vi "kalman transmit and receive state updates.vi"(7 "min photons to update":u32, 8 "update z":bool, 9 "update y":bool, 10 "update x":bool, 11 "3-axis PV tracking state":T2) -> (0 "Timed Out?":bool, 2 "num kalmans queued":u16, 3 "3-axis PV tracking state out":T2, 4 "kalman to host":cluster{"Kalman State":T1, "Kalman Update":bool})   [LabVIEW 2010]
uses:
  kalman 3-axis state.ctl
  integrating single axis kalman state.ctl
  <vilib>/rvi/DataTransferAndStorage/Container/XNode/niFpgaContainer.xnode
  <vilib>/rvi/FIFO/Fifo_Resource/nirvififoEmulationSetSize.vi
  <vilib>/rvi/DataTransferAndStorage/Container/Common/niFpgaContainerGetUniqueNameForEmu.vi
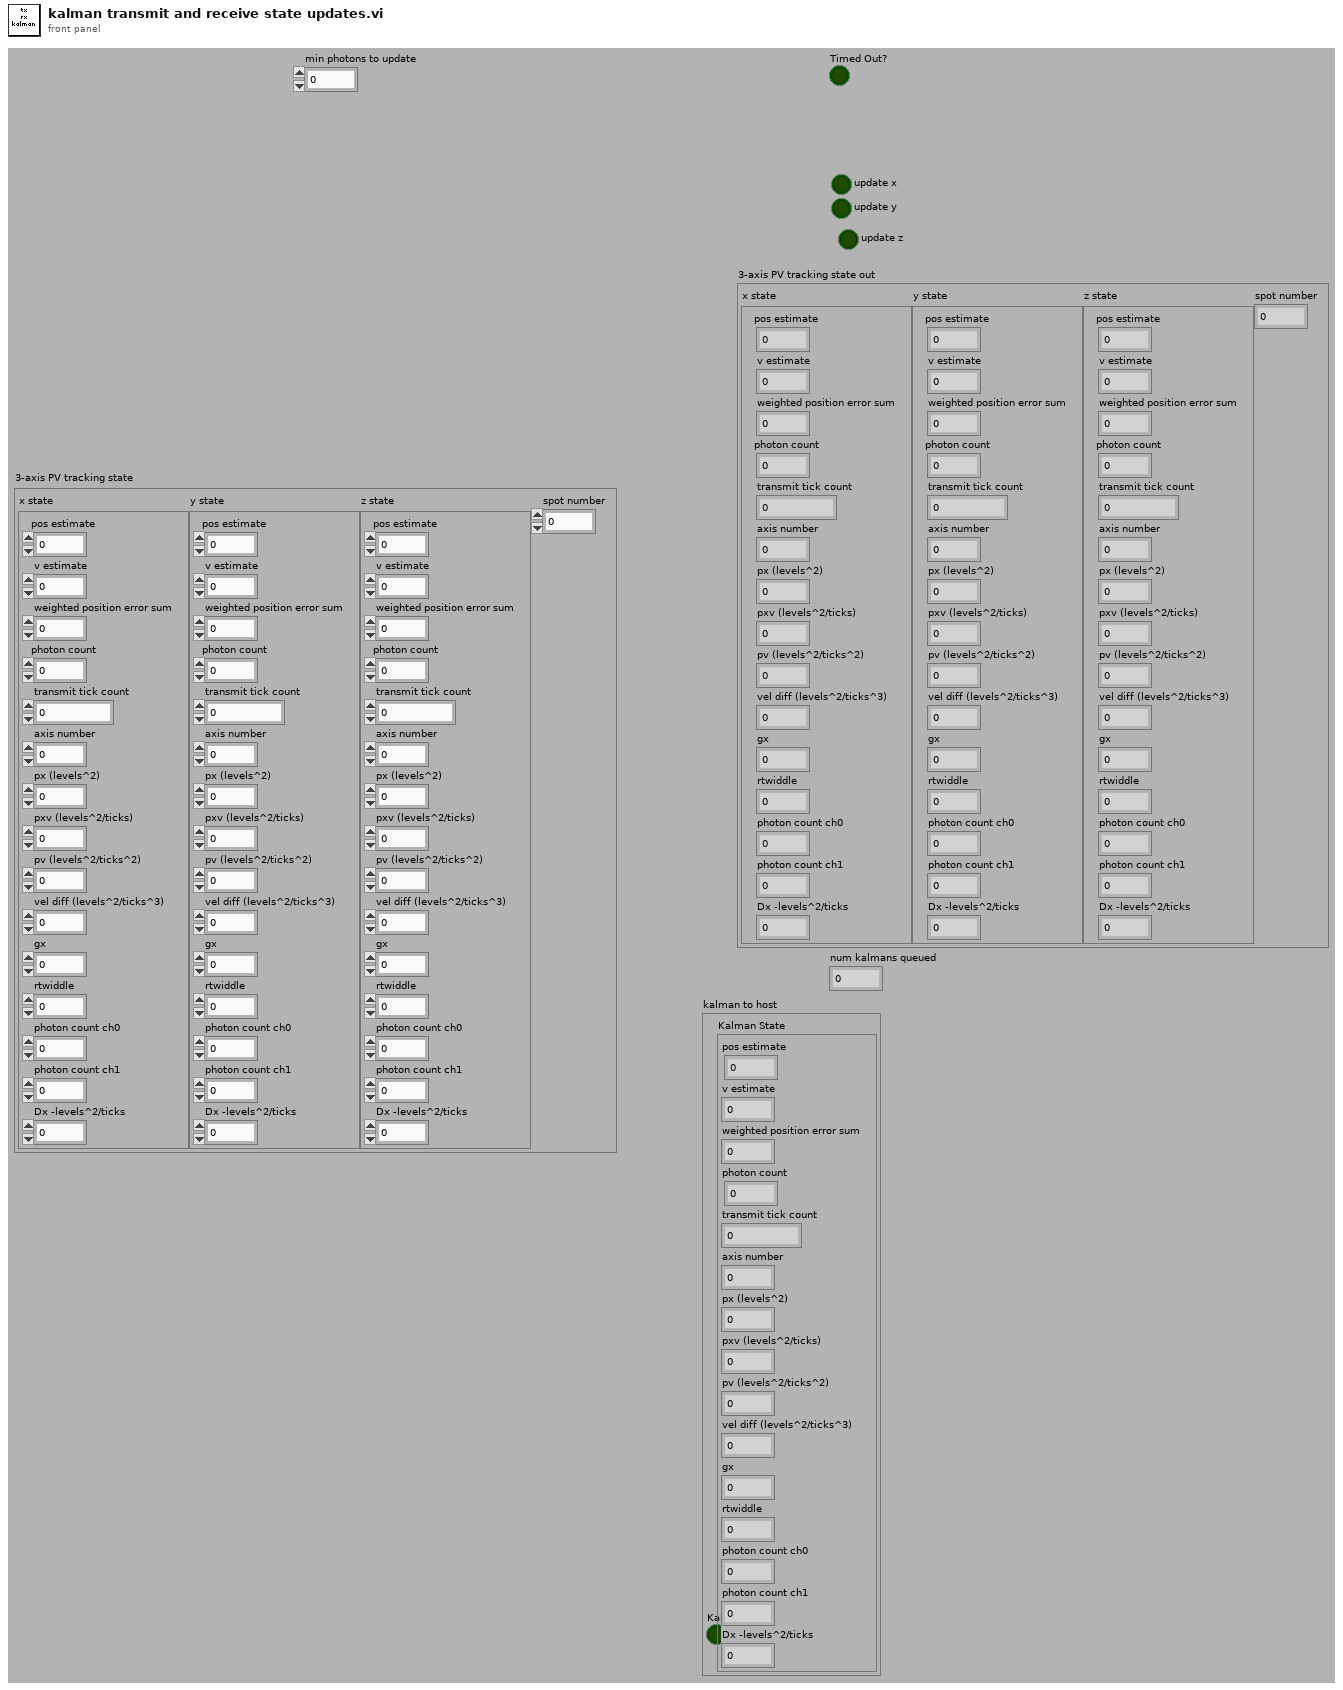
[diagram p1: front panel]
types:
  T1 = typedef "integrating single axis kalman state.ctl" = cluster{"pos estimate":fxp<+/-,32,16>, "v estimate":fxp<+/-,16,0>, "weighted position error sum":fxp<+/-,32,32>, "photon count":u32, "transmit tick count":u32, "axis number":u8, "px (levels^2)":fxp<+,32,19>, "pxv (levels^2/ticks)":fxp<+,32,2>, "pv (levels^2/ticks^2)":fxp<+,32,-14>, "vel diff (levels^2/ticks^3)":fxp<+,24,-22>, "gx":fxp<+,16,8>, "rtwiddle":fxp<+,16,26>, "photon count ch0":u32, "photon count ch1":u32, "Dx -levels^2/ticks":fxp<+,32,19>}
  T2 = typedef "kalman 3-axis state.ctl" = cluster{"x state":T1, "y state":T1, "z state":T1, "spot number":u8}
  T3 = cluster{"pos estimate":fxp<+/-,32,16>, "v estimate":fxp<+/-,16,0>, "weighted position error sum":fxp<+/-,32,32>, "photon count":u32, "transmit tick count":u32, "axis number":u8, "px (levels^2)":fxp<+,32,19>, "pxv (levels^2/ticks)":fxp<+,32,2>, "pv (levels^2/ticks^2)":fxp<+,32,-14>, "vel diff (levels^2/ticks^3)":fxp<+,24,-22>, "gx":fxp<+,16,8>, "rtwiddle":fxp<+,16,26>, "photon count ch0":u32, "photon count ch1":u32, "Dx - for pos only k-f":fxp<+,32,19>}
  T4 = cluster{"Element":cluster{"pos estimate":fxp<+/-,32,16>, "v estimate":fxp<+/-,16,0>, "weighted position error sum":fxp<+/-,32,32>, "photon count":u32, "transmit tick count":u32, "axis number":u8, "px (levels^2)":fxp<+,32,19>, "pxv (levels^2/ticks)":fxp<+,32,2>, "pv (levels^2/ticks^2)":fxp<+,32,-14>, "vel diff (levels^2/ticks^3)":fxp<+,24,-22>, "gx":fxp<+,16,8>, "rtwiddle":fxp<+,16,26>, "photon count ch0":u32, "photon count ch1":u32, "Dx - for pos only k-f":fxp<+,32,19>}, bool}
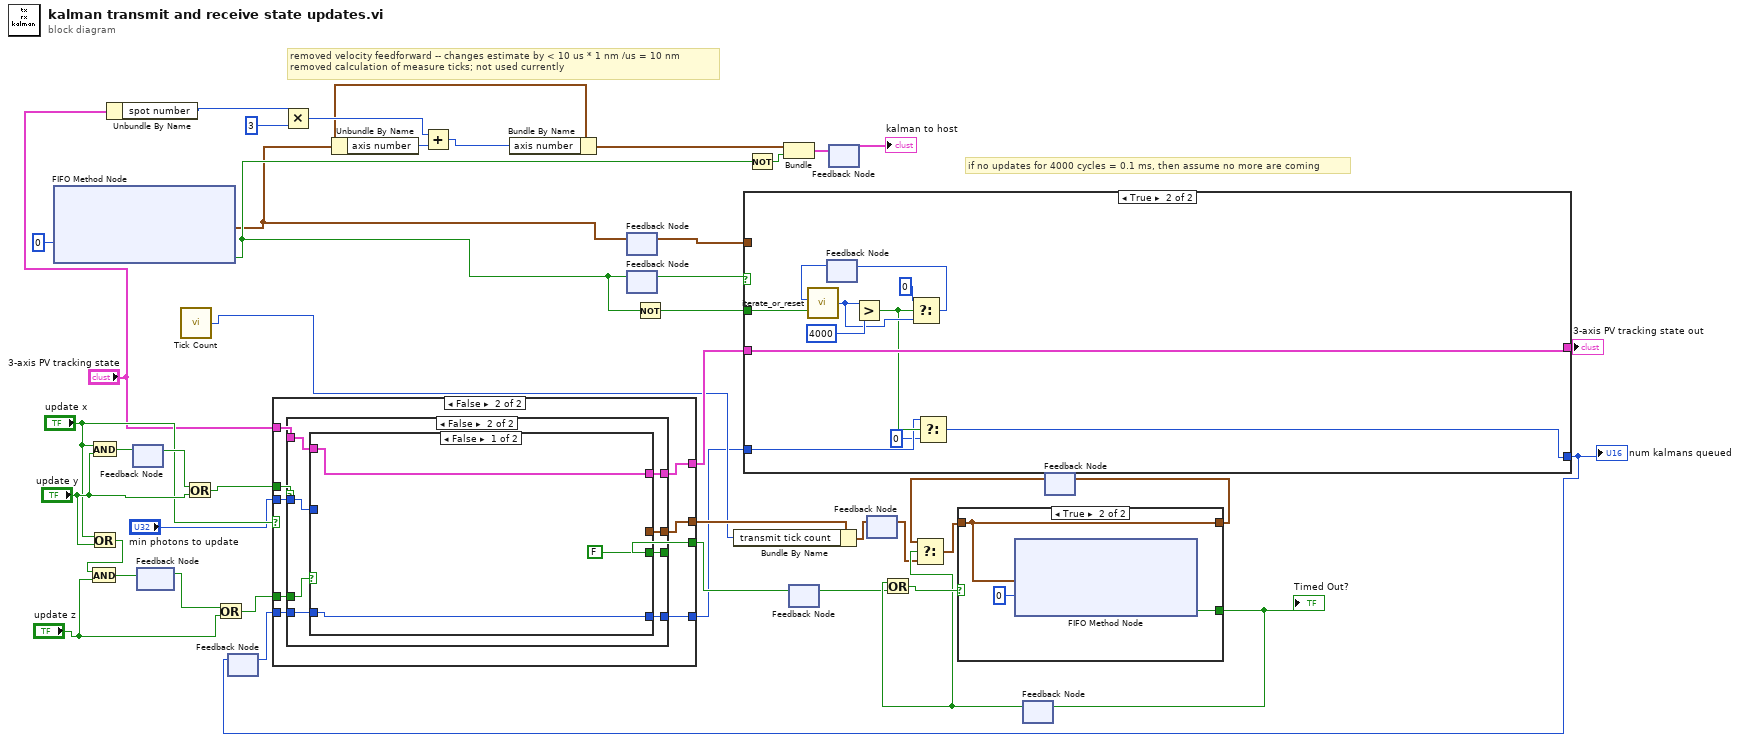
[diagram p0: block diagram]
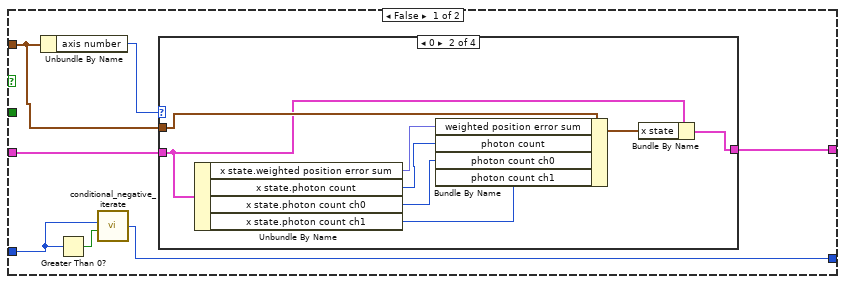
[diagram p2: hidden frame]
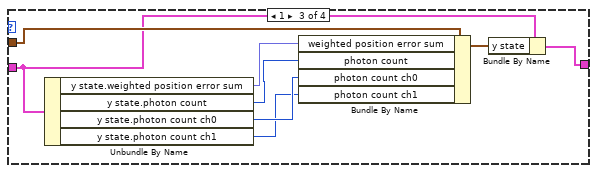
[diagram p4: hidden frame]
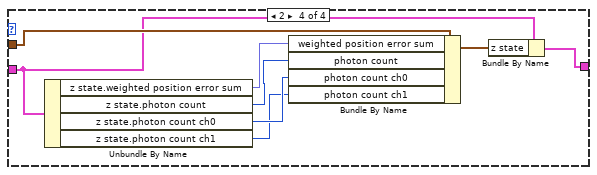
[diagram p5: hidden frame]
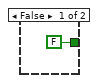
[diagram p6: hidden frame]
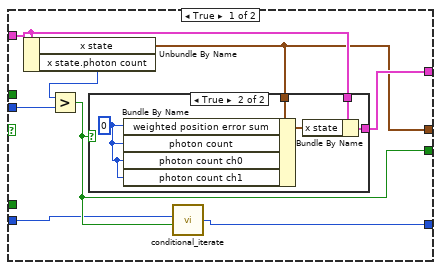
[diagram p7: hidden frame]
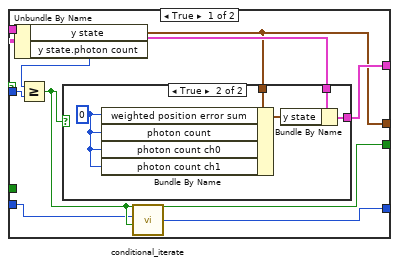
[diagram p9: hidden frame]
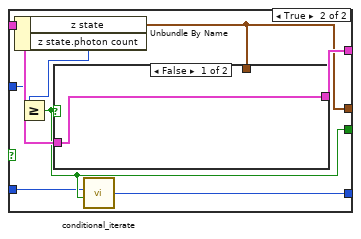
[diagram p11: hidden frame]
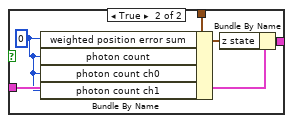
[diagram p12: hidden frame]
diagram:
  # "if no updates for 4000 cycles = 0.1 ms, then assume no more are coming"
  # "removed velocity feedforward -- changes estimate by < 10 us * 1 nm /us = 10 nm\nremoved calculation of measure ticks; not used currently"
  n1 = xnode ("FIFO Method Node")("Timeout"=0) -> ("Element"=w1:T3, "Timed Out?"=w10:bool)  [unwired: 1 in, 1 out]
  n2 = And(x="update x", y="update y") -> (x .and. y?=w44:bool)
  n3 = Or(x="update x", y="update y") -> (x .or. y?=w41:bool)
  n4 = And(x=w41, y="update z") -> (x .and. y?=w40:bool)
  n5 = Unbundle By Name("3-axis PV tracking state") -> ("spot number"=w2:u8)
  n6 = feedback-in #1(w44) -> ()
  n7 = feedback #1() -> (w43:bool)  [unwired: 1 in]
  n8 = feedback #2() -> (w39:bool)  [unwired: 1 in]
  n9 = feedback-in #2(w40) -> ()
  n10 = call "Tick Count"() -> ("Tick Count(Ticks)"=w21:u32)
  n11 = Or(x=w43, y="update y") -> (x .or. y?=w36:bool)
  n12 = Or(x=w39, y="update z") -> (x .or. y?=w35:bool)
  n13 = feedback #3() -> (w13:u16)  [unwired: 1 in]
  n14 = case shown="False" "update x" {
    tunnel: "3-axis PV tracking state" -> [w52 w67]
    tunnel: [w51 w66] -> w26
    tunnel: [w50 w65] -> w33
    tunnel: [w47 w64] -> w34
    tunnel: w36 -> [_ w63]
    tunnel: w35 -> [_ w62]
    tunnel: "min photons to update" -> [w48 w61]
    tunnel: [w45 w60] -> w14
    tunnel: w13 -> [w46 w59]
    frame True {
      n15 = Unbundle By Name(w52) -> ("x state"=w50:T1, "x state.photon count"=w49:u32)
      n16 = Greater?(x=w49, y=w48) -> (0:w47:bool)
      n17 = case shown="True" w47 {
        tunnel: w52 -> [w53 w57]
        tunnel: [w53 w56] -> w51
        tunnel: w50 -> [_ w55]
        frame False {
        }
        frame True {
          w54 = i16 0
          n18 = Bundle By Name(cluster=w55, "weighted position error sum"=w54, "photon count"=w54, "photon count ch0"=w54, "photon count ch1"=w54) -> (w58:T1)
          n19 = Bundle By Name(cluster=w57, "x state"=w58) -> (w56:T2)
        }
      }
      n20 = call "conditional_iterate.vi"("iterate?"=w47, "number in"=w46) -> ("number out"=w45:u16)  [unwired: 4 in]
    }
    frame False {
      n21 = case shown="False" w63 {
        tunnel: w67 -> [w75 w89]
        tunnel: [w74 w88] -> w66
        tunnel: [w73 w87] -> w65
        tunnel: [w70 w86] -> w64
        tunnel: w62 -> [_ w85]
        tunnel: w61 -> [w72 w84]
        tunnel: [w68 w83] -> w60
        tunnel: w59 -> [w69 w82]
        frame True {
          n22 = Unbundle By Name(w75) -> ("y state"=w73:T1, "y state.photon count"=w71:u32)
          n23 = Greater Or Equal?(x=w71, y=w72) -> (x >= y?=w70:bool)
          n24 = case shown="True" w70 {
            tunnel: w75 -> [w76 w80]
            tunnel: [w76 w79] -> w74
            tunnel: w73 -> [_ w78]
            frame False {
            }
            frame True {
              w77 = i16 0
              n25 = Bundle By Name(cluster=w78, "weighted position error sum"=w77, "photon count"=w77, "photon count ch0"=w77, "photon count ch1"=w77) -> (w81:T1)
              n26 = Bundle By Name(cluster=w80, "y state"=w81) -> (w79:T2)
            }
          }
          n27 = call "conditional_iterate.vi"("iterate?"=w70, "number in"=w69) -> ("number out"=w68:u16)  [unwired: 4 in]
        }
        frame False {
          n28 = case shown="False" w85 {
            tunnel: w89 -> [w92 w100]
            tunnel: [w92 w99] -> w88
            tunnel: [_ w98] -> w87
            tunnel: [FALSE w95] -> w86
            tunnel: w84 -> [_ w97]
            tunnel: [w90 w94] -> w83
            tunnel: w82 -> [w90 w93]
            frame False {
            }
            frame True {
              n29 = Unbundle By Name(w100) -> ("z state"=w98:T1, "z state.photon count"=w96:u32)
              n30 = Greater Or Equal?(x=w96, y=w97) -> (x >= y?=w95:bool)
              n31 = case shown="False" w95 {
                tunnel: w100 -> [w101 w105]
                tunnel: [w101 w104] -> w99
                tunnel: w98 -> [_ w103]
                frame False {
                }
                frame True {
                  w102 = i16 0
                  n32 = Bundle By Name(cluster=w103, "weighted position error sum"=w102, "photon count"=w102, "photon count ch0"=w102, "photon count ch1"=w102) -> (w106:T1)
                  n33 = Bundle By Name(cluster=w105, "z state"=w106) -> (w104:T2)
                }
              }
              n34 = call "conditional_iterate.vi"("iterate?"=w95, "number in"=w93) -> ("number out"=w94:u16)  [unwired: 4 in]
            }
          }
        }
      }
    }
  }
  n35 = Multiply(x=w2, y=u8 3) -> (x*y=w5:u8)
  n36 = Unbundle By Name(w1) -> ("axis number"=w7:u8)
  n37 = Add(x=w5, y=w7) -> (x+y=w4:u8)
  n38 = Bundle By Name(cluster=w1, "axis number"=w4) -> (w8:T3)
  n39 = feedback-in #4(w1) -> ()
  n40 = feedback #4() -> (w18:T3)  [unwired: 1 in]
  n41 = feedback #5() -> (w11:bool)  [unwired: 1 in]
  n42 = feedback-in #5(w10) -> ()
  n43 = Not(x=w10) -> (.not. x?=w9:bool)
  n44 = Bundle By Name(cluster=w33, "transmit tick count"=w21) -> (w22:T1)
  n45 = case shown="True" w11 {
    tunnel: w18 -> [w110 _]
    tunnel: w26 -> [w112 w149]
    tunnel: [w111 w149] -> w25
    tunnel: w14 -> [w109 w141]
    tunnel: [w107 w139] -> w12
    tunnel: w9 -> [_ w148]
    frame False {
      n46 = Unbundle By Name(w110) -> ("axis number"=w113:u8)
      n47 = Greater Than 0?(x=w109) -> (x > 0?=w108:bool)
      n48 = call "conditional_negative_iterate.vi"("iterate?"=w108, "number in"=w109) -> ("number out"=w107:u16)  [unwired: 4 in]
      n49 = case shown="0" w113 {
        tunnel: w112 -> [w114 w119 w127 w135]
        tunnel: [w114 w117 w125 w133] -> w111
        tunnel: w110 -> [_ w122 w130 w138]
        frame Default {
        }
        frame 0 {
          n50 = Unbundle By Name(w119) -> ("x state.weighted position error sum"=w121:fxp<+/-,32,32>, "x state.photon count"=w120:u32, "x state.photon count ch0"=w116:u32, "x state.photon count ch1"=w115:u32)
          n51 = Bundle By Name(cluster=w122, "weighted position error sum"=w121, "photon count"=w120, "photon count ch0"=w116, "photon count ch1"=w115) -> (w118:T3)
          n52 = Bundle By Name(cluster=w119, "x state"=w118) -> (w117:T2)
        }
        frame 1 {
          n53 = Unbundle By Name(w127) -> ("y state.weighted position error sum"=w129:fxp<+/-,32,32>, "y state.photon count"=w128:u32, "y state.photon count ch0"=w124:u32, "y state.photon count ch1"=w123:u32)
          n54 = Bundle By Name(cluster=w130, "weighted position error sum"=w129, "photon count"=w128, "photon count ch0"=w124, "photon count ch1"=w123) -> (w126:T3)
          n55 = Bundle By Name(cluster=w127, "y state"=w126) -> (w125:T2)
        }
        frame 2 {
          n56 = Unbundle By Name(w135) -> ("z state.weighted position error sum"=w137:fxp<+/-,32,32>, "z state.photon count"=w136:u32, "z state.photon count ch0"=w132:u32, "z state.photon count ch1"=w131:u32)
          n57 = Bundle By Name(cluster=w138, "weighted position error sum"=w137, "photon count"=w136, "photon count ch0"=w132, "photon count ch1"=w131) -> (w134:T3)
          n58 = Bundle By Name(cluster=w135, "z state"=w134) -> (w133:T2)
        }
      }
    }
    frame True {
      n59 = feedback #6() -> (w147:u16)  [unwired: 1 in]
      n60 = call "iterate_or_reset.vi"("iterate?"=w148, "number in"=w147) -> ("number out"=w145:u16)  [unwired: 4 in]
      n61 = Greater?(x=w145, y=u16 4000) -> (0:w142:bool)
      n62 = Select(t=u16 0, s=w142, f=w145) -> (s? t:f=w143:u16)
      n63 = feedback-in #6(w143) -> ()
      n64 = Select(t=w141, s=w142, f=u16 0) -> (s? t:f=w139:u16)
    }
  }
  "3-axis PV tracking state out" <- w25
  "num kalmans queued" <- w12
  n65 = feedback-in #3(w12) -> ()
  n66 = Not(x=w10) -> (.not. x?=w16:bool)
  n67 = Bundle("Element"=w8, w16) -> (w17:T4)  [unwired: 1 in]
  n68 = feedback-in #7(w34) -> ()
  n69 = feedback #7() -> (w19:bool)  [unwired: 1 in]
  n70 = feedback-in #8(w17) -> ()
  n71 = feedback #8() -> (→"kalman to host":T4)  [unwired: 1 in]
  n72 = feedback-in #9(w22) -> ()
  n73 = feedback #9() -> (w20:T1)  [unwired: 1 in]
  n74 = feedback #10() -> (w29:bool)  [unwired: 1 in]
  n75 = Or(x=w29, y=w19) -> (x .or. y?=w30:bool)
  n76 = feedback #11() -> (w28:T1)  [unwired: 1 in]
  n77 = Select(t=w28, s=w29, f=w20) -> (s? t:f=w32:T1)
  n78 = case shown="True" w30 {
    tunnel: w32 -> [_ w151]
    tunnel: [FALSE ("Timed Out?") w152] -> w31
    tunnel: [_ w151] -> w23
    frame False {
    }
    frame True {
      n79 = xnode ("FIFO Method Node")("Element"=w151, "Timeout"=0) -> ("Timed Out?"=w152:bool)  [unwired: 1 in, 1 out]
    }
  }
  "Timed Out?" <- w31
  n80 = feedback-in #10(w31) -> ()
  n81 = feedback-in #11(w23) -> ()
